vi "Dashboard Main.vi"() -> ()   [LabVIEW 2014]
uses:
  <vilib>/event_ctls.llb/eventvkey.ctl
  <vilib>/Rock Robotics/WPI/Dashboard/WPI_DashboardLogging Global.vi
  <vilib>/Rock Robotics/Network Tables/SD Read Number.vi
  <vilib>/Rock Robotics/Network Tables/SD Write Boolean.vi
  <vilib>/Rock Robotics/Network Tables/SD Write Number.vi
  <vilib>/Utility/config.llb/Write Key (String).vi
  <vilib>/Utility/config.llb/Write Key (I32).vi
  <vilib>/Utility/config.llb/NI_LVConfig.lvlib
panel:
  out "Controls Open 2":bool
  in  "TCP":refnum<k5>
  in  "Rec Mode":enum32{"Stop", "Record", "Playback"}(radio)
  in  "Vision":u16(ring) items=["Camera Off", "USB Camera SW", "USB Camera HW", "IP Camera"]
  out "Camera IP":string
  out "Image Message":string="Timeout in Camera Communications"
  in  "Dashboard Tab":T1(tab)
  in  "?":bool
  in  "?":bool
  in  "Camera Settings":T2={"Frame Rate"=30, "Compression"=30, "Size"=1} {"Frame Rate" scale=1.0..30.0; "Size" items=["640x480", "320x240", "160x120"]}
  out "MotorChart R":cluster{"Numeric":dbl, "Numeric":dbl}(graph)
  out "MotorChart L":T3(graph)
  out "MotorSliders R":cluster{"MotorSlide1":dbl, "MotorSlide2":dbl} {"MotorSlide2" scale=-1.0..1.0 scale format="%#_2e"; "MotorSlide1" scale=-1.0..1.0 scale format="%#_2e"}
  out "MotorSliders L":T4 {"MotorSlide4 2" scale=0.0..14.0 scale format="%#_2e"; "MotorSlide2" scale=-1.0..1.0 scale format="%#_2e"; "MotorSlide1" scale=-1.0..1.0 scale format="%#_2e"}
  out "Gyro":dbl(knob) scale=0.0..360.0
  out "JS1 Z":dbl(slide) scale=-1.0..1.0 scale format="%#_2e"
  out "JS1 Graph":cluster{"X":dbl, "Y":dbl}[](graph)
  out "JS1 Buttons":T5
  out "JS2 Z":dbl(slide) scale=-1.0..1.0 scale format="%#_2e"
  out "JS2 Graph":cluster{"X":dbl, "Y":dbl}[](graph)
  out "JS2 Buttons":T5
  out "Mode":T6(ring)=enum."Auto Disabled"
  in  "DB Camera Config":bool
  out "fps":dbl format="%#.1g"
  out "Mbps":dbl format="%#.1g"
  out "Mbps 2":bool
  in  "DB/String 9":string
  in  "DB/String 8":string
  in  "DB/String 7":string
  in  "DB/String 6":string
  in  "DB/String 5":string
  in  "DB/String 4":string
  in  "DB/String 3":string
  in  "DB/String 2":string
  in  "DB/String 1":string
  in  "DB/String 0":string
  in  "DB/Slider 0":dbl(slide) scale=0.0..5.0
  in  "DB/Slider 1":dbl(slide) scale=0.0..5.0
  in  "DB/Slider 2":dbl(slide) scale=0.0..5.0
  in  "DB/Slider 3":dbl(slide) scale=0.0..5.0
  out "DB/LED 3":bool
  out "DB/LED 2":bool
  out "DB/LED 1":bool
  out "DB/LED 0":bool
  in  "DB/Button 3":bool
  in  "DB/Button 2":bool
  in  "DB/Button 1":bool
  in  "DB/Button 0":bool caption="New Name"
  in  "Auto Encoder Set Point":dbl=10.0
  out "Right Potentiometer":dbl
  out "Left Potentiometer":dbl
  in  "Test Slider":dbl(slide) scale=0.0..100.0 scale format="%#_3g"
  in  "On/Off":bool caption="Solenoid"
  in  "Test Name":u16(ring) items=["Select the test to run...", "Example Test", "-------------------------------", "List of tests is built in robot code.", "Replace with your own automated tests."]
  in  "Test Tree":string(tree)
  in  "Motor":cluster{"Value":dbl, "Enable":bool} {"Value" scale=-1.0..1.0 scale format="%#_3g"}
  out "Progress":T7 {"Test Progress" scale=0.0..100.0}
  in  "Rev/Fwd":cluster{"Forward":bool, "Reverse":bool}
  in  "Test Ring":u16(ring) items=["Monochrome", "Color"]
  in  "Listbox":i32(listbox)
  out "Tree":string(tree)
  out "Camera Image":T8(plugin-control)
  out "Boolean":bool
  out "Controls Open":bool
  # "Left"
  # "Front"
  # "Right"
  # "Battery"
  # "This tab is a great place for autonomous settings and robot-specific values.\nPlace controls and indicators inside this tab and match name to\nDashboard Variables on robot. You can also delete this comment."
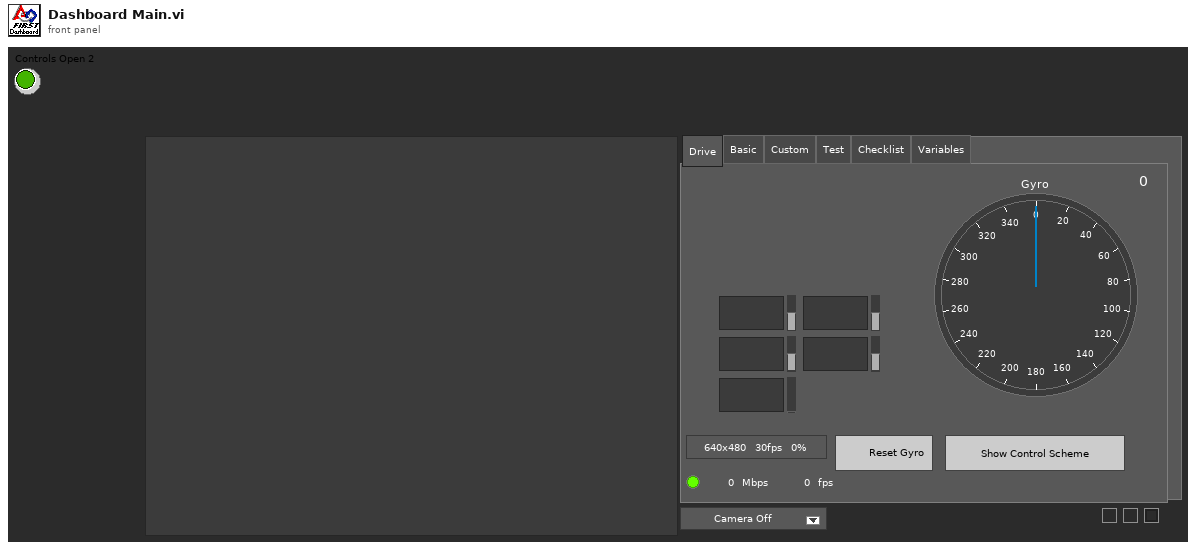
[diagram p1: front panel]
types:
  T1 = enum32{"Drive", "Basic", "Custom", "Test", "Checklist", "Variables"}
  T2 = cluster{"Frame Rate":i32, "Compression":i32, "Size":u16}
  T3 = cluster{"Numeric":dbl, "Numeric":dbl, "Battery V":dbl}
  T4 = cluster{"MotorSlide1":dbl, "MotorSlide2":dbl, "MotorSlide4 2":dbl}
  T5 = cluster{bool, bool, bool, bool, bool, bool, bool, bool, bool, bool, bool, bool}
  T6 = enum8{"Tele-Op Disabled", "Tele-Op Enabled", "Auto Disabled", "Auto Enabled", "Test Disabled", "Test Enabled", "Disconnected", "No Code", "E-Stop"}
  T7 = cluster{"Test Progress":u8, "Test Progress Text":string}
  T8 = typedef "IMAQ Image.ctl" = refnum<image>
  T9 = typedef "Image Type" = u32
  T10 = cluster{"Camera Image":refnum<vi>, "Dashboard Tab":refnum<vi>, "Boolean":refnum<vi>, "Vision":refnum<vi>, "Rec Mode":refnum<vi>, "Test Slider":refnum<vi>, "On/Off ":refnum<vi>, "Test Ring":refnum<vi>, "Rev/Fwd":refnum<vi>, "Test Name":refnum<vi>, "Motor":refnum<vi>, "Progress":refnum<vi>, "CheckList":refnum<vi>, "Tree":refnum<vi>, "Test Tree":refnum<vi>}
  T11 = cluster{"Error Strings":string, "Disable Counts":cluster{u16, u16}, "Rail Faults":cluster{u16, u16, u16}, "Robot IP":string, "DB Mode":u8, "Event Info":cluster{"Name":string, "Type":u8, "Number":u16, "Replay":u8}, "Camera Addr":string}
  T12 = cluster{"Storage":cluster{"Disk Free":u64, "RAM Block":u32, "RAM free":u32}, "CPU Utilization":cluster{"CPU % ISR":sgl, "CPU % Time Crit":sgl, "CPU % Timed Str":sgl, "CPU % High":sgl, "CPU % Above":sgl, "CPU % Normal":sgl, "CPU % Low":sgl}, "CAN":cluster{"% Bus Utilization":sgl, "Bus Off Cnt":u32, "TX_FIFO Full Cnt":u32, "Receive Error Cnt":u8, "Transmit Error Cnt":u8}, "HID":cluster{"HID Outputs":u32, "Rumble Low":u16, "Rumble High":u16}[]}
  T13 = cluster{"Status bits":cluster{"Test Mode":bool, "Autonomous":bool, "Enabled":bool, "Code Start":bool, "Brownout":bool, "Reserved 2":bool, "Reserved 3":bool, "E-Stop":bool}, "Code Trace":cluster{"Disabled":bool, "TeleOp":bool, "Auto":bool, "Test":bool}, "Controller Type":enum16{"unknown", "cRIO", "roboRio"}, "Code?":enum16{"unknown", "noCode", "code"}, "Battery V":dbl}
  T14 = cluster{"Control Bits":cluster{"TestMode":bool, "Autonomous":bool, "Enabled":bool, "FMS Present":bool, bool, bool, bool, "E-Stop":bool}, "Team Station ":u8, "Countdown":sgl, "Joystick Values":cluster{"Axes":dbl[], "Buttons":bool[], "POVs":i16[]}[]}
  T15 = cluster{"Axes":dbl[], "Buttons":bool[], "POVs":i16[]}[]
  T16 = cluster{"Axes":dbl[], "Buttons":bool[], "POVs":i16[]}
  T17 = cluster{"Buttons[0]":bool, "Buttons[1]":bool, "Buttons[2]":bool, "Buttons[3]":bool, "Buttons[4]":bool, "Buttons[5]":bool, "Buttons[6]":bool, "Buttons[7]":bool, "Buttons[8]":bool, "Buttons[9]":bool, "Buttons[10]":bool, "Buttons[11]":bool}
  T18 = typedef "NI_LVConfig.lvlib/Config Data RefNum.ctl" = refnum<k1>
  T19 = cluster{"Operation":enum16{"Update", "Clear"}, "Color Box":u32}[]
  T20 = typedef "eventvkey.ctl" = enum16{"ASCII", "Enter", "Return", "Shift", "Ctrl", "Alt", "Cmd", "Opt", "Caps", "NumLock", "Clear", "Break", "Up", "Down", "Left", "Right", "Insert", "Delete", "Home", "End", "PageUp", "PageDown", "Escape", "Help", "Pause", "ScrollLock", "F1", "F2", "F3", "F4", "F5", "F6", "F7", "F8", "F9", "F10", "F11", "F12", "F13", "F14", "F15", "F16", "F17", "F18", "F19", "F20", "F21", "F22", "F23", "F24", "Play", "VolumeUp", "VolumeDown", "Mute", "Two Byte Char"}
  T21 = cluster{"Image Size":bool, "Image Type":bool, "Pixel Value":bool, "ROI Information":bool, "Zoom Factor":bool}
  T22 = enum8{"Enabled", "Disabled", "Disabled and Grayed Out"}
  T23 = cluster{"Operation":enum16{"Update", "Clear"}, "Color Box":u32}
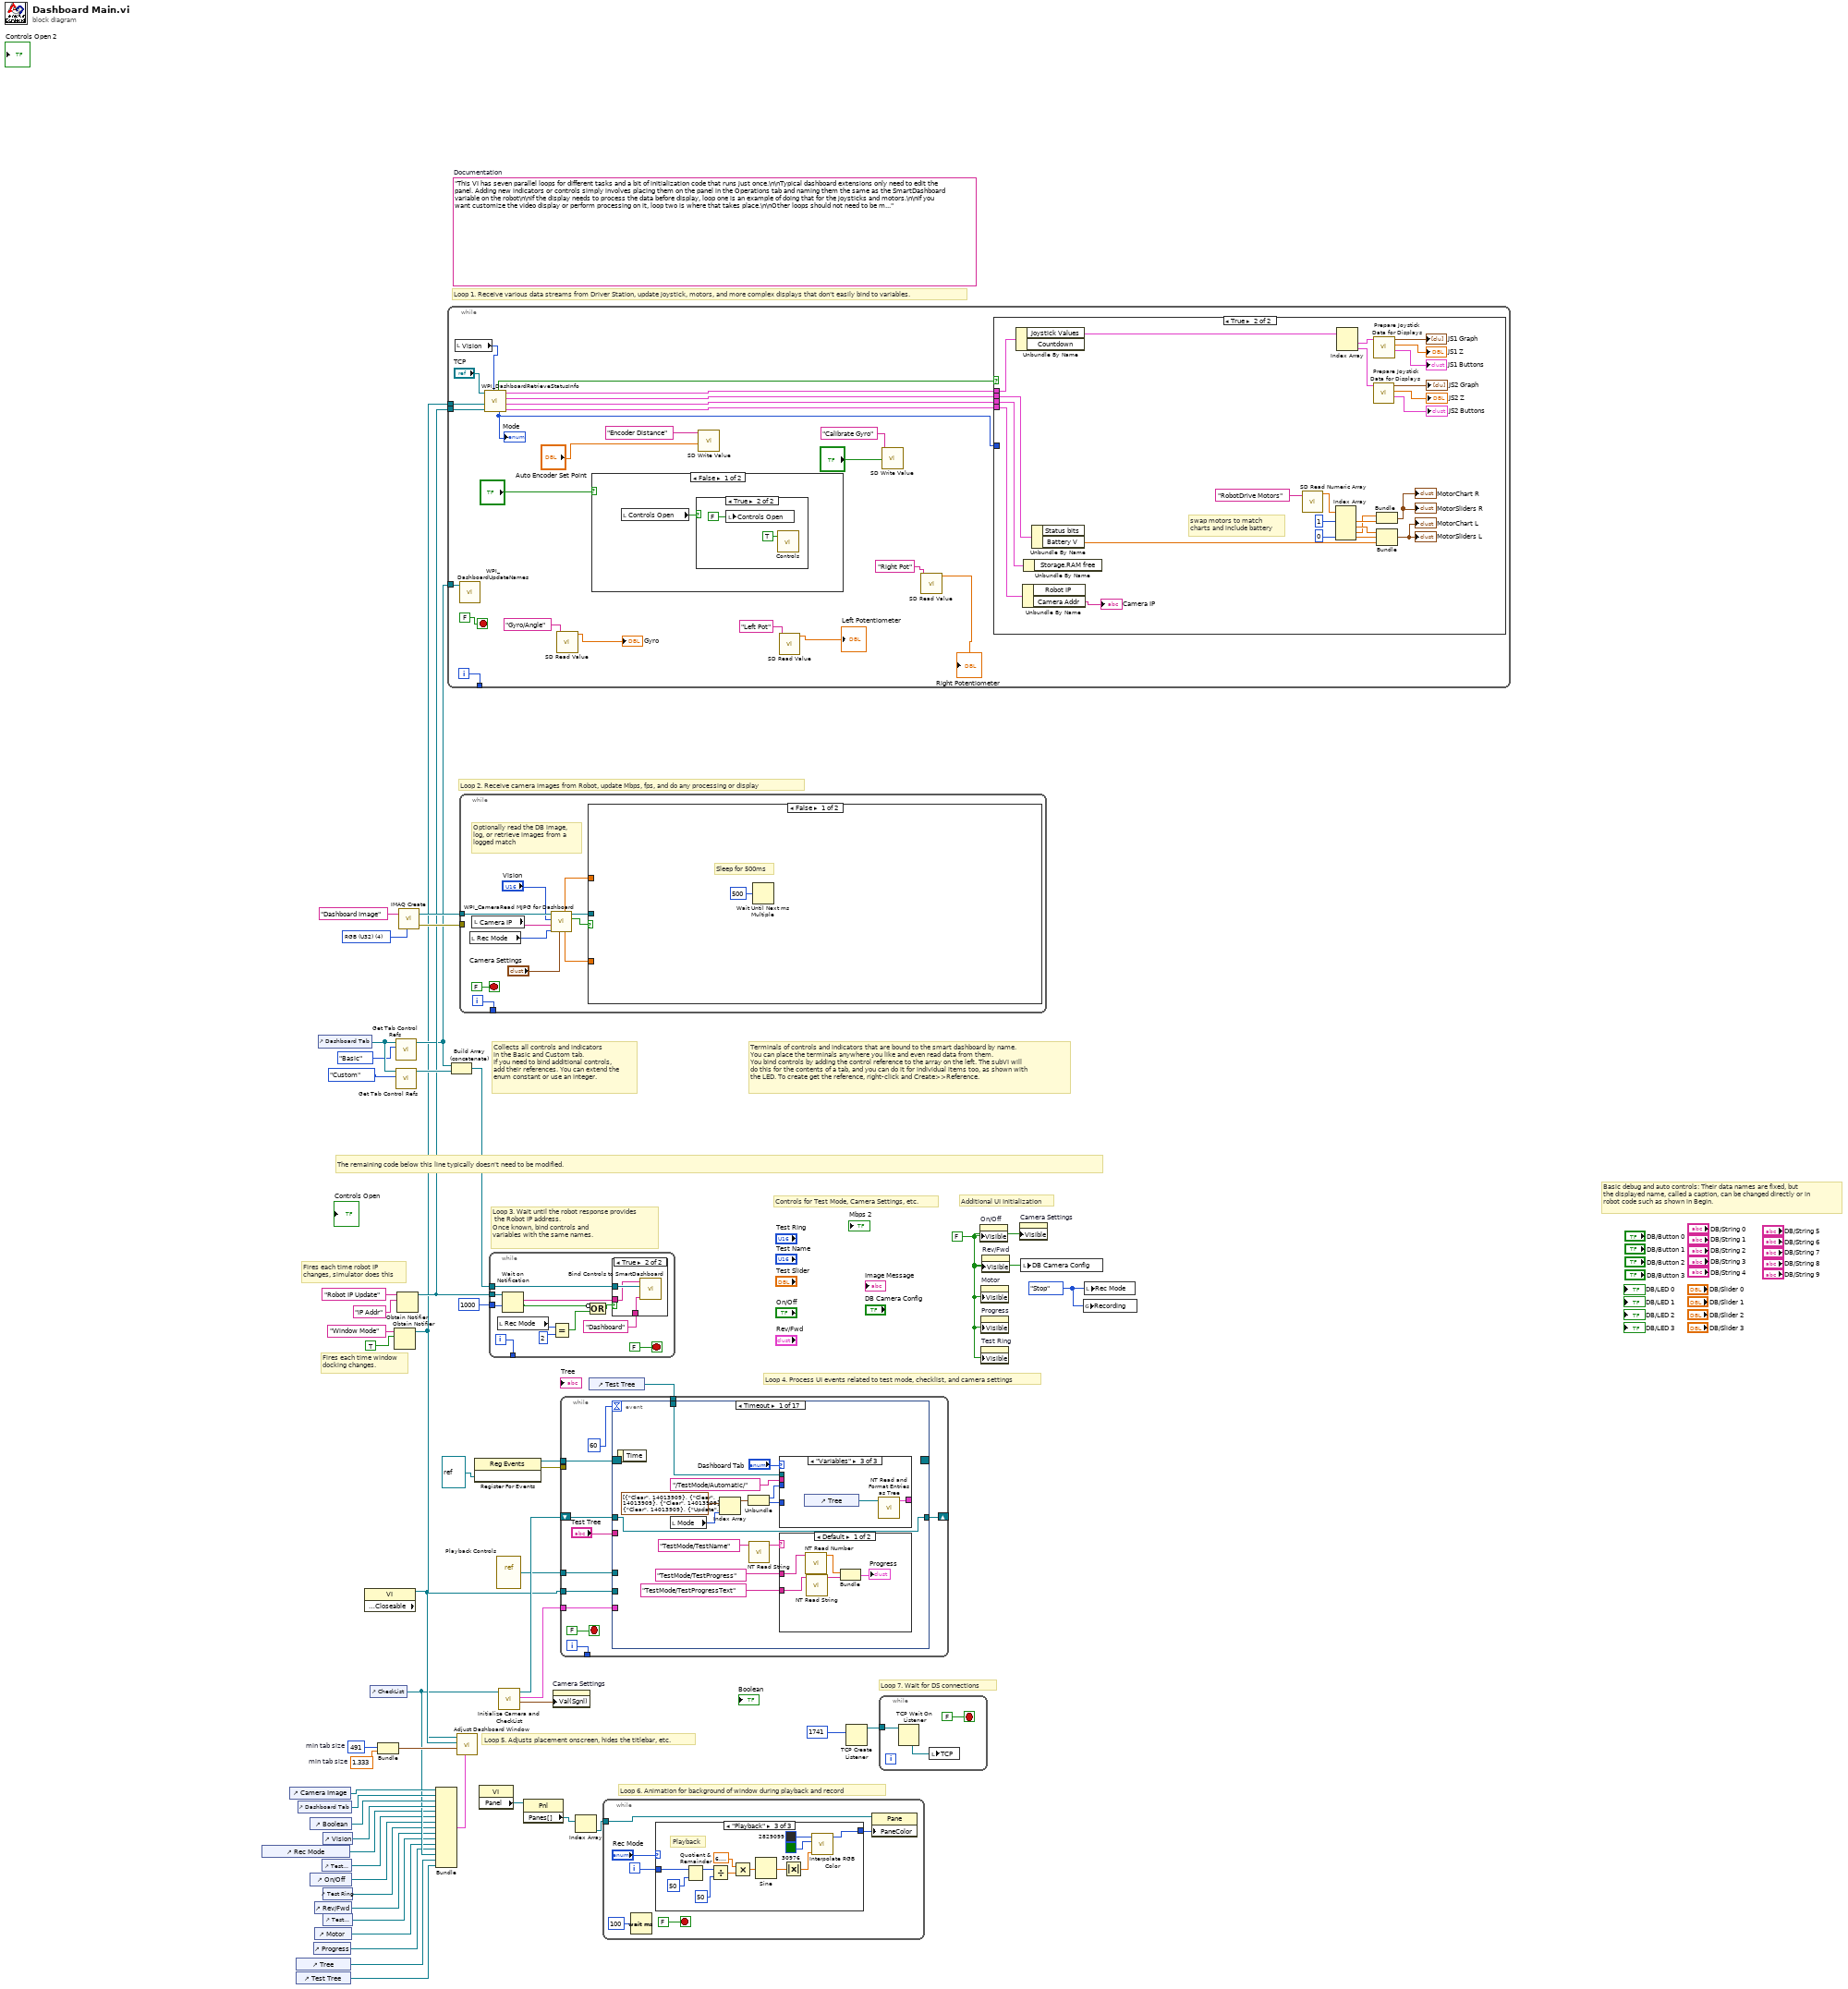
[diagram p0: block diagram]
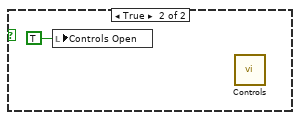
[diagram p3: hidden frame]
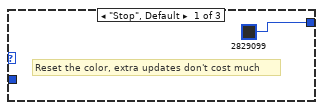
[diagram p5: hidden frame]
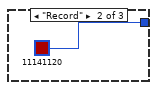
[diagram p6: hidden frame]
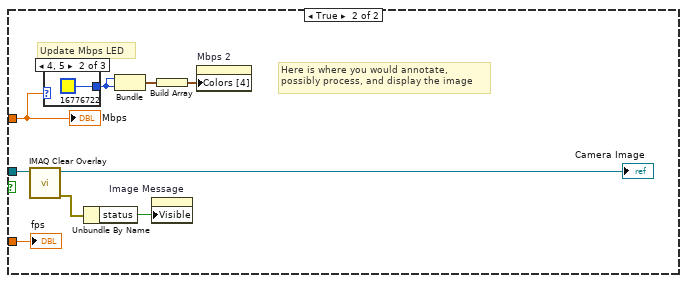
[diagram p8: hidden frame]
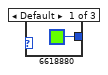
[diagram p9: hidden frame]
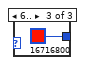
[diagram p10: hidden frame]
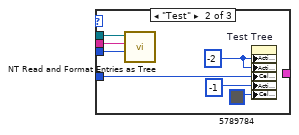
[diagram p12: hidden frame]
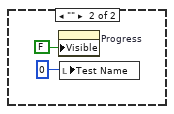
[diagram p13: hidden frame]
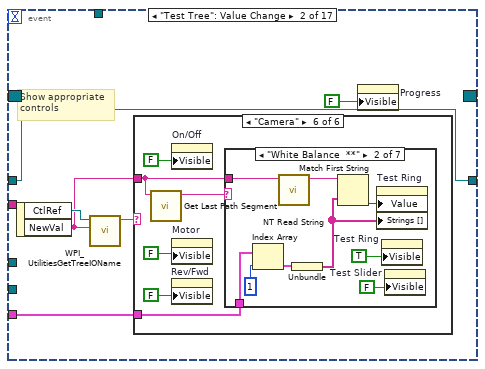
[diagram p14: hidden frame]
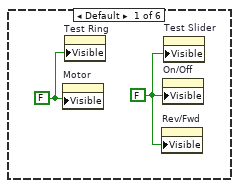
[diagram p15: hidden frame]
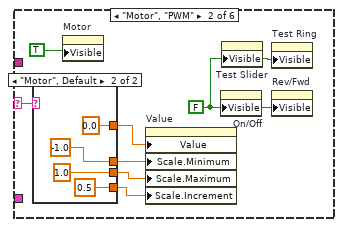
[diagram p16: hidden frame]
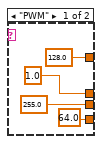
[diagram p17: hidden frame]
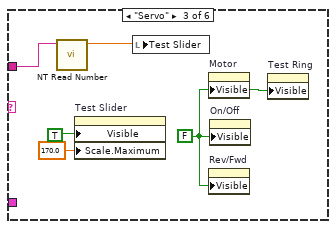
[diagram p18: hidden frame]
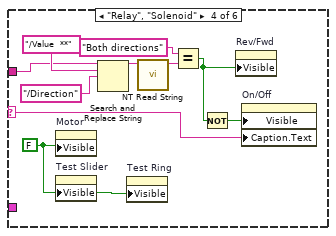
[diagram p19: hidden frame]
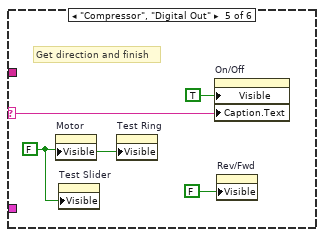
[diagram p20: hidden frame]
diagram:
  w24 = 491  # min tab size
  w23 = 1.333  # min tab size
  w32 = enum32{"Stop", "Record", "Playback"}."Stop" ("Rec Mode")
  w6 = FALSE ("Visible")
  (unwired) "This VI has seven parallel loops for different tasks and a bit of initialization code that runs just once.\n\nTypical dashboard extensions only need to edit the panel. Adding new indicators or controls simply involves placing them on the panel in the Operations tab and naming them the same as the SmartDashboard variable on the robot\n\nIf the display needs to process the data before display, loop one is an example of doing that for the joysticks and motors.\n\nIf you want customize the video display or perform processing on it, loop two is where that takes place.\n\nOther loops should not need to be modified. They are pretty standard, and document the task they perform."  # Documentation
  w52 = T9 4 items=["Grayscale (U8)", "Grayscale (I16)", "Grayscale (SGL)", "Complex (CSG)", "RGB (U32)", "HSL (U32)", "RGB (U64)"] ("Image Type")
  # "Loop 7. Wait for DS connections"
  # "Basic debug and auto controls: Their data names are fixed, but\nthe displayed name, called a caption, can be changed directly or in\nrobot code such as shown in Begin."
  # "Controls for Test Mode, Camera Settings, etc."
  # "Additional UI Initialization"
  # "Loop 6. Animation for background of window during playback and record"
  # "Fires each time robot IP\nchanges, simulator does this"
  # "Fires each time window\ndocking changes."
  # "Collects all controls and indicators\nin the Basic and Custom tab.\nIf you need to bind additional controls,\nadd their references. You can extend the\nenum constant or use an integer."
  # "The remaining code below this line typically doesn't need to be modified."
  # "Loop 4. Process UI events related to test mode, checklist, and camera settings"
  # "Terminals of controls and indicators that are bound to the smart dashboard by name.\nYou can place the terminals anywhere you like and even read data from them.\nYou bind controls by adding the control reference to the array on the left. The subVI will\ndo this for the contents of a tab, and you can do it for individual items too, as shown with\nthe LED. To create get the reference, right-click and Create>>Reference."
  # "Loop 3. Wait until the robot response provides\n the Robot IP address.\nOnce known, bind controls and\nvariables with the same names."
  # "Loop 5. Adjusts placement onscreen, hides the titlebar, etc."
  # "Loop 1. Receive various data streams from Driver Station, update joystick, motors, and more complex displays that don't easily bind to variables."
  # "Loop 2. Receive camera images from Robot, update Mbps, fps, and do any processing or display"
  n1 = control-ref of="Rec Mode"() -> (w12:refnum<vi>)
  n2 = control-ref of="Camera Image"() -> (w27:refnum<vi>)
  n3 = control-ref of="Tree"() -> (w16:refnum<vi>)
  n4 = control-ref of="Test Tree"() -> (w15:refnum<vi>)
  n5 = control-ref of="Dashboard Tab"() -> (w26:refnum<vi>)
  n6 = control-ref of="Boolean"() -> (w21:refnum<vi>)
  n7 = control-ref of="On/Off"() -> (w10:refnum<vi>)
  n8 = control-ref of="Progress"() -> (w7:refnum<vi>)
  n9 = control-ref of="Rev/Fwd"() -> (w8:refnum<vi>)
  n10 = control-ref of="Motor"() -> (w13:refnum<vi>)
  n11 = control-ref of="Dashboard Tab"() -> (w30:refnum<vi>)
  n12 = control-ref of="Test Slider"() -> (w11:refnum<vi>)
  n13 = control-ref of="Vision"() -> (w25:refnum<vi>)
  n14 = control-ref of="Test Ring"() -> (w9:refnum<vi>)
  n15 = control-ref of="Test Name"() -> (w14:refnum<vi>)
  n16 = property class="VI" props=["Front Panel.Closeable"]() -> (reference out=w31:refnum<vi>)  [unwired: 2 in, 2 out]
  n17 = control-ref of="CheckList"() -> (w17:refnum<vi>)
  n18 = Bundle("min tab size"=w24, "min tab size"=w23) -> (w22:cluster{"min tab size":i32, "min tab size":dbl})  [unwired: 1 in]
  n19 = Obtain Notifier(name (unnamed)="Window Mode", notification data type=TRUE) -> (notifier out=w3:refnum<notifier>)  [unwired: 2 in, 2 out]
  n20 = call <vilib>:"Get Tab Control Refs.vi"("Page Index"=T1."Basic" ("Dashboard Tab"), "TabControl in"=w30) -> ("ControlsOnPage"=w4:refnum<vi>[])  [unwired: 9 in]
  n21 = call <vilib>:"Get Tab Control Refs.vi"("Page Index"=T1."Custom" ("Dashboard Tab"), "TabControl in"=w30) -> ("ControlsOnPage"=w29:refnum<vi>[])  [unwired: 9 in]
  n22 = Obtain Notifier(name (unnamed)="Robot IP Update", notification data type="IP Addr" ("name (unnamed)")) -> (notifier out=w5:refnum<notifier>)  [unwired: 2 in, 2 out]
  n23 = call "IMAQ Create"("Image Name"="Dashboard Image", "Image Type"=w52) -> ("New Image"=w50:T8, "error out"=w49:errorcluster)  [unwired: 2 in, 1 out]
  n24 = Bundle("Camera Image"=w27, "Dashboard Tab"=w26, "Boolean"=w21, "Vision"=w25, "Rec Mode"=w12, "Test Slider"=w11, "On/Off"=w10, "Test Ring"=w9, "Rev/Fwd"=w8, "Test Name"=w14, "Motor"=w13, "Progress"=w7, "CheckList"=w17, "Tree"=w16, "Test Tree"=w15) -> (w18:T10)  [unwired: 1 in]
  n25 = while {
    tunnel: [w75] -> _
    tunnel: w5 -> [w69]
    tunnel: w4 -> [w68]
    tunnel: w3 -> [w64]
    i -> [w75]
    stop <- FALSE stop-if-true
    n26 = local read "Vision"() -> (w66:u16)
    n27 = call <vilib>:"WPI_DashboardUpdateNames.vi"("Controls on Tab"=w68) -> ()  [unwired: 11 in]
    n28 = call <vilib>:"WPI_DashboardRetrieveStatusInfo.vi"("Vision"=w66, "Binding Refnum"=w69, "Window Mode Notifier"=w64, "TCP Cnx"="TCP") -> ("Power and Errors"=w70:T11, "Robot Metrics"=w73:T12, "Status Info"=w74:T13, "Control Info"=w71:T14, "Robot Mode"=w67:T6, "Process?"=w72:bool)  [unwired: 2 in]
    "Mode" <- w67
    n29 = call-poly <vilib>:"SD Read Value.vi"("Name"="Gyro/Angle") -> ("Numeric"=→"Gyro":dbl)  [unwired: 8 in, 2 out]
    n30 = case shown="False" "?" {
      frame False {
        n31 = local read "Controls Open"() -> (w77:bool)
        n32 = case shown="True" w77 {
          frame False {
          }
          frame True {
            n33 = local write "Controls Open"(FALSE ("Controls Open")) -> ()
            n34 = call "Controls.vi"("Close"=TRUE) -> ()  [unwired: 11 in]
          }
        }
      }
      frame True {
        n35 = local write "Controls Open"(TRUE) -> ()
        n36 = call "Controls.vi"() -> ()  [unwired: 12 in]
      }
    }
    n37 = call-poly <vilib>:"SD Write Value.vi"("Numeric"="Auto Encoder Set Point", "Name"="Encoder Distance") -> ()  [unwired: 8 in, 2 out]
    n38 = call-poly <vilib>:"SD Read Value.vi"("Name"="Left Pot") -> ("Numeric"=→"Left Potentiometer":dbl)  [unwired: 8 in, 2 out]
    n39 = call-poly <vilib>:"SD Write Value.vi"("Boolean"="?", "Name"="Calibrate Gyro") -> ()  [unwired: 8 in, 2 out]
    n40 = call-poly <vilib>:"SD Read Value.vi"("Name"="Right Pot") -> ("Numeric"=→"Right Potentiometer":dbl)  [unwired: 8 in, 2 out]
    n41 = case shown="True" w72 {
      tunnel: w74 -> [_ w105]
      tunnel: w73 -> [_ w104]
      tunnel: w71 -> [_ w103]
      tunnel: w70 -> [_ w102]
      tunnel: w67 -> [_ _]
      frame False {
      }
      frame True {
        # "swap motors to match\ncharts and include battery"
        n42 = Unbundle By Name(w103) -> ("Joystick Values"=w90:T15)  [unwired: 1 out]
        n43 = Unbundle By Name(w102) -> ("Camera Addr"=→"Camera IP":string)  [unwired: 1 out]
        n44 = Unbundle By Name(w104) -> ()  [unwired: 1 out]
        n45 = Unbundle By Name(w105) -> ("Battery V"=w91:dbl)  [unwired: 1 out]
        n46 = call <vilib>:"SD Read Numeric Array.vi"("Name"="RobotDrive Motors") -> ("Numeric Array"=w93:dbl[])  [unwired: 8 in, 2 out]
        n47 = Index Array(array=w93, index #1=1, index #4=0) -> (element #1=w97:dbl, element #2=w98:dbl, element #3=w96:dbl, element #4=w101:dbl)  [unwired: 2 in]
        n48 = Index Array(array=w90) -> (element #1=w89:T16, element #2=w84:T16)  [unwired: 2 in]
        n49 = call "Prepare Joystick Data for Displays.vi"("Joystick Values"=w84) -> ("Buttons"=→"JS2 Buttons":T17, "Z Axis"=→"JS2 Z":dbl, "Cartesian Data"=→"JS2 Graph":cluster{"X axis":dbl, "X axis":dbl}[])  [unwired: 8 in]
        n50 = call "Prepare Joystick Data for Displays.vi"("Joystick Values"=w89) -> ("Buttons"=→"JS1 Buttons":T17, "Z Axis"=→"JS1 Z":dbl, "Cartesian Data"=→"JS1 Graph":cluster{"X axis":dbl, "X axis":dbl}[])  [unwired: 8 in]
        n51 = Bundle("Numeric"=w96, "Numeric"=w97) -> (→"MotorChart R" →"MotorSliders R":cluster{"Numeric":dbl, "Numeric":dbl})  [unwired: 1 in]
        n52 = Bundle("Numeric"=w98, "Numeric"=w101, "Battery V"=w91) -> (→"MotorChart L" →"MotorSliders L":T3)  [unwired: 1 in]
      }
    }
  }
  n53 = Build Array (concatenate)(w4, w29) -> (w28:refnum<vi>[])
  n54 = call "Adjust Dashboard Window.vi"("Sizing Refnums"=w18, "Size Constraints"=w22, "VI"=w31, "Notifier in"=w3) -> ()  [unwired: 8 in]
  n55 = while {
    tunnel: w50 -> [w114]
    tunnel: w49 -> [_]
    tunnel: [w115] -> _
    i -> [w115]
    stop <- FALSE stop-if-true
    # "Optionally read the DB image,\nlog, or retrieve images from a\nlogged match"
    n56 = local read "Rec Mode"() -> (w108:enum32{"Stop", "Record", "Playback"})
    n57 = local read "Camera IP"() -> (w106:string)
    n58 = call <vilib>:"WPI_CameraRead MJPG for Dashboard.vi"("Camera Settings"="Camera Settings", "Rec Mode"=w108, "Camera IP"=w106, "Camera Mode"="Vision", "Refnum in"=w114) -> ("Active"=w112:bool, "Refnum out"=w113:T8, "FPS"=w111:dbl, "Bandwidth (Mbps)"=w110:dbl)  [unwired: 3 in]
    n59 = case shown="False" w112 {
      tunnel: w113 -> [_ w121]
      tunnel: w110 -> [_ w120]
      tunnel: w111 -> [_ w118]
      frame False {
        # "Sleep for 500ms"
        n60 = Wait Until Next ms Multiple(millisecond multiple=u32 500) -> ()  [unwired: 1 out]
      }
      frame True {
        # "Here is where you would annotate,\npossibly process, and display the image"
        # "Update Mbps LED"
        n61 = call "IMAQ Clear Overlay"("Image"=w121) -> ("error out"=w125:errorcluster, "Image Out"=→"Camera Image":T8)  [unwired: 2 in, 7 out]
        n62 = case shown="4, 5" w120 {
          tunnel: [u32 6618880 ("Color Box") u32 16776722 ("Color Box") u32 16716800 ("Color Box")] -> w122
          frame Default {
          }
          frame 4, 5 {
          }
          frame 6.. {
          }
        }
        n63 = Unbundle By Name(w125) -> ("status"=w126:bool)
        n64 = Bundle("Color Box"=w122, "Color Box"=w122) -> (w124:cluster{"Color Box":u32, "Color Box":u32})  [unwired: 1 out]
        n65 = property on="Image Message" class="Str"("Visible"=w126) -> ()  [unwired: 2 in, 2 out]
        n66 = Build Array(w124) -> (w123:cluster{"Color Box":u32, "Color Box":u32}[])
        n67 = property on="Mbps 2" class="Bool (strict)"("Colors [4]"=w123) -> ()  [unwired: 2 in, 2 out]
        "Mbps" <- w120
        "fps" <- w118
      }
    }
  }
  n68 = register-events(refnum<vi> refnum) -> (reference out=w36:refnum<event-registration>, error out=w35:errorcluster)  [unwired: 2 in]
  n69 = property class="VI"() -> ("Panel"=w39:refnum<vi>)  [unwired: 2 in, 2 out]
  n70 = while {
    tunnel: w28 -> [w141]
    tunnel: w5 -> [w139]
    tunnel: [w137] -> _
    tunnel: u32 1000 ("milliseconds to wait") -> [w136]
    i -> [w137]
    stop <- FALSE stop-if-true
    n71 = local read "Rec Mode"() -> (w132:enum32{"Stop", "Record", "Playback"})
    n72 = Wait on Notification(notifier=w139, timeout in ms (-1)=w136) -> (notification=w138:string, timed out?=w134:bool)  [unwired: 2 in, 2 out]
    n73 = Equal?(x=w132, y=u16 2 ("Rec Mode")) -> (x = y?=w133:bool)
    n74 = Compound Arithmetic op=OR(invert w134, w133) -> (w135:bool)
    n75 = case shown="True" w135 {
      tunnel: w141 -> [_ w144]
      tunnel: w138 -> [_ w143]
      tunnel: "Dashboard" -> [_ w142]
      frame False {
      }
      frame True {
        n76 = call <vilib>:"Bind Controls to SmartDashboard.vi"("Client Name"=w142, "Bound Control Refs"=w144, "Server IP Address"=w143) -> ()  [unwired: 9 in]
      }
    }
  }
  n77 = vi-ref "Playback Controls.vi"() -> (w37:refnum<vi>)
  n78 = call "Initialize Camera and CheckList.vi"("ListBox in"=w17) -> ("Cluster"=w43:cluster{"value":i32, "value":i32, "index":i32}, "Array"=w44:cluster{string[]}[], "File Refnum"=w42:T18)  [unwired: 8 in]
  n79 = property class="Pnl"(reference=w39) -> ("Panes[]"=w40:refnum<vi>[])  [unwired: 1 in, 2 out]
  n80 = property on="Camera Settings" class="Clust (strict)"("Val(Sgnl)"=w43) -> ()  [unwired: 2 in, 2 out]
  n81 = Index Array(array=w40) -> (element=w38:refnum<vi>)  [unwired: 1 in]
  n82 = control-ref of="Test Tree"() -> (w41:refnum<vi>)
  n83 = while {
    tunnel: w44 -> [w152]
    shift-right: [w151] -> _
    shift-left: w42 -> [w150]
    tunnel: [w149] -> _
    tunnel: w41 -> [w148]
    tunnel: w37 -> [w147]
    tunnel: w36 -> [w146]
    tunnel: w35 -> [_]
    tunnel: w31 -> [w145]
    i -> [w149]
    stop <- FALSE stop-if-true
    n84 = event shown="[0] Timeout" {
      selector: w146 -> [_ _ _ _ _ _ _ _ _ _ _ _ _ _ _ _ _]
      dyn-events: [_ _ _ _ _ _ _ _ _ _ _ _ _ w390 _ _ _] -> _
      timeout: u32 60 ("milliseconds to wait") -> [_ _ _ _ _ _ _ _ _ _ _ _ _ _ _ _ _]
      tunnel: w148 -> [w164 _ _ _ _ _ _ _ _ _ _ _ _ _ _ _ _]
      tunnel: "Test Tree" -> [_ _ _ _ _ _ _ _ w359 w367 w369 w373 w381 _ _ _ _]
      tunnel: w152 -> [_ w186 _ _ _ _ w323 w353 _ _ _ _ _ _ _ _ _]
      tunnel: [w160 w185 w284 w289 w297 w309 w322 w346 w358 w365 w368 w372 w380 w392 w406 w407 w417] -> w151
      tunnel: w150 -> [w160 w185 w284 w289 w297 w309 w321 w346 w358 w365 w368 w372 w380 w392 w406 w407 w417]
      tunnel: w147 -> [_ _ _ _ _ _ _ _ _ _ _ _ _ w393 _ w410 _]
      tunnel: w145 -> [_ _ _ _ _ _ _ _ _ _ _ _ _ w388 _ _ _]
      event Timeout {
        n85 = event-data() -> ()  [unwired: 1 in, 1 out]
        n86 = local read "Mode"() -> (w163:T6)
        n87 = Index Array(array=T19 [{"Operation"=enum."Clear", "Color Box"=14013909}, {"Operation"=enum."Clear", "Color Box"=14013909}, {"Operation"=enum."Clear", "Color Box"=14013909}, {"Operation"=enum."Clear", "Color Box"=14013909}, {"Operation"=enum."Update", "Color Box"=14013909}, {"Operation"=enum."Update", "Color Box"=16777215}, {"Operation"=enum."Clear", "Color Box"=14013909}, {"Operation"=enum."Clear", "Color Box"=14013909}, {"Operation"=enum."Clear", "Color Box"=14013909}], index=w163) -> (element=w158:T23)
        n88 = Unbundle(w158) -> ("Operation"=w157:enum16{"Update", "Clear"}, "Color Box"=w156:u32)
        n89 = call <vilib>:"NT Read String.vi"("Name"="TestMode/TestName") -> ("String"=w167:string)  [unwired: 9 in, 1 out]
        n90 = case shown="\"Variables\"" "Dashboard Tab" {
          tunnel: w164 -> [_ w175 _]
          tunnel: "/TestMode/Automatic/" ("Name Pattern") -> [_ w174 _]
          tunnel: w157 -> [_ w173 _]
          tunnel: [_ _ w177] -> _
          tunnel: w156 -> [_ w169 _]
          frame "Custom", Default {
          }
          frame "Test" {
            w172 = -2 ("Active Item:Row Number")
            n91 = call <vilib>:"NT Read and Format Entries as Tree.vi"("Operation"=w173, "Name Pattern"=w174, "Tree Refnum"=w175) -> ()  [unwired: 7 in, 2 out]
            n92 = property on="Test Tree" class="Tree (strict)"("Active Item Row Number"=w172, "ActiveColNum"=w172, "CellBG"=w169, "Active Item Row Number"=-1 ("Active Item:Row Number"), "CellBG"=u32 5789784 ("Color Box")) -> ()  [unwired: 2 in, 2 out]
          }
          frame "Variables" {
            n93 = control-ref of="Tree"() -> (w176:refnum<vi>)
            n94 = call <vilib>:"NT Read and Format Entries as Tree.vi"("Tree Refnum"=w176) -> ("Formatted Strings"=w177:cluster{"Name":string, "Value":string}[])  [unwired: 9 in, 1 out]
          }
        }
        n95 = case shown="Default" w167 {
          tunnel: "TestMode/TestProgress" ("Name") -> [w179 _]
          tunnel: "TestMode/TestProgressText" ("Name") -> [w178 _]
          frame Default {
            n96 = call <vilib>:"NT Read Number.vi"("Name"=w179) -> ("Numeric"=w180:dbl)  [unwired: 9 in, 1 out]
            n97 = call <vilib>:"NT Read String.vi"("Name"=w178) -> ("String"=w181:string)  [unwired: 9 in, 1 out]
            n98 = Bundle("Numeric"=w180, "String"=w181) -> (→"Progress":cluster{"Numeric":dbl, "String":string})  [unwired: 1 in]
          }
          frame "" {
            n99 = property on="Progress" class="Clust (strict)"("Visible"=FALSE) -> ()  [unwired: 2 in, 2 out]
            n100 = local write "Test Name"(u16 0) -> ()
          }
        }
      }
      event "Test Tree": Value Change {
        # "Show appropriate\ncontrols"
        n101 = event-data() -> ("CtlRef"=w189:refnum<vi>, "NewVal"=w187:string)  [unwired: 1 in]
        n102 = call <vilib>:"WPI_UtilitiesGetTreeIOName.vi"("NewVal"=w187, "TreeControl in"=w189) -> ("I/O Name"=w190:string)  [unwired: 9 in]
        n103 = case shown="\"Camera\"" w190 {
          selector: w190 -> [_ w197 _ w215 w224 _]
          tunnel: w187 -> [_ _ w212 w214 _ w231]
          tunnel: w186 -> [_ _ _ _ _ w230]
          frame Default {
            w192 = FALSE ("Visible")
            w191 = FALSE ("Visible")
            n104 = property on="Motor" class="Clust (strict)"("Visible"=w191) -> ()  [unwired: 2 in, 2 out]
            n105 = property on="Test Ring" class="Ring (strict)"("Visible"=w191) -> ()  [unwired: 2 in, 2 out]
            n106 = property on="Rev/Fwd" class="Clust (strict)"("Visible"=w192) -> ()  [unwired: 2 in, 2 out]
            n107 = property on="On/Off" class="Bool (strict)"("Visible"=w192) -> ()  [unwired: 2 in, 2 out]
            n108 = property on="Test Slider" class="Slide (strict)"("Visible"=w192) -> ()  [unwired: 2 in, 2 out]
          }
          frame "Motor", "PWM" {
            w198 = FALSE ("Visible")
            n109 = case shown="\"Motor\", Default" w197 {
              tunnel: [1.0 ("Value") -1.0 ("Value")] -> w196
              tunnel: [255.0 ("Value") 1.0 ("Value")] -> w195
              tunnel: [128.0 ("Value") 0.0 ("Value")] -> w194
              tunnel: [64.0 ("Value") 0.5 ("Value")] -> w193
              frame "PWM" {
              }
              frame "Motor", Default {
              }
            }
            n110 = property on="Motor" class="Clust (strict)"("Visible"=TRUE) -> ()  [unwired: 2 in, 2 out]
            n111 = property on="Value" class="Slide (strict)"("Value"=w194, "Scale.Minimum"=w196, "Scale.Maximum"=w195, "Scale.Increment"=w193) -> ()  [unwired: 2 in, 2 out]
            n112 = property on="On/Off" class="Bool (strict)"("Visible"=w198) -> ()  [unwired: 2 in, 2 out]
            n113 = property on="Test Slider" class="Slide (strict)"("Visible"=w198) -> ()  [unwired: 2 in, 2 out]
            n114 = property on="Test Ring" class="Ring (strict)"("Visible"=w198) -> ()  [unwired: 2 in, 2 out]
            n115 = property on="Rev/Fwd" class="Clust (strict)"("Visible"=w198) -> ()  [unwired: 2 in, 2 out]
          }
          frame "Servo" {
            w210 = FALSE ("Visible")
            n116 = call <vilib>:"NT Read Number.vi"("Name"=w212) -> ("Numeric"=w211:dbl)  [unwired: 9 in, 1 out]
            n117 = property on="Test Slider" class="Slide (strict)"("Visible"=TRUE, "Scale.Maximum"=170.0 ("Scale.Range:Maximum")) -> ()  [unwired: 2 in, 2 out]
            n118 = local write "Test Slider"(w211) -> ()
            n119 = property on="Motor" class="Clust (strict)"("Visible"=w210) -> ()  [unwired: 2 in, 2 out]
            n120 = property on="Rev/Fwd" class="Clust (strict)"("Visible"=w210) -> ()  [unwired: 2 in, 2 out]
            n121 = property on="On/Off" class="Bool (strict)"("Visible"=w210) -> ()  [unwired: 2 in, 2 out]
            n122 = property on="Test Ring" class="Ring (strict)"("Visible"=w210) -> ()  [unwired: 2 in, 2 out]
          }
          frame "Relay", "Solenoid" {
            w213 = FALSE ("Visible")
            n123 = property on="Motor" class="Clust (strict)"("Visible"=w213) -> ()  [unwired: 2 in, 2 out]
            n124 = property on="Test Slider" class="Slide (strict)"("Visible"=w213) -> ()  [unwired: 2 in, 2 out]
            n125 = Search and Replace String(input string=w214, search string="/Value  **", replace string="/Direction") -> (result string=w220:string)  [unwired: 5 in, 3 out]
            n126 = property on="Test Ring" class="Ring (strict)"("Visible"=w213) -> ()  [unwired: 2 in, 2 out]
            n127 = call <vilib>:"NT Read String.vi"("Name"=w220) -> ("String"=w218:string)  [unwired: 9 in, 1 out]
            n128 = Equal?(x="Both directions", y=w218) -> (x = y?=w216:bool)
            n129 = Not(x=w216) -> (.not. x?=w217:bool)
            n130 = property on="Rev/Fwd" class="Clust (strict)"("Visible"=w216) -> ()  [unwired: 2 in, 2 out]
            n131 = property on="On/Off" class="Bool (strict)"("Visible"=w217, "Caption.Text"=w215) -> ()  [unwired: 2 in, 2 out]
          }
          frame "Compressor", "Digital Out" {
            w223 = FALSE ("Visible")
            # "Get direction and finish"
            n132 = property on="Motor" class="Clust (strict)"("Visible"=w223) -> ()  [unwired: 2 in, 2 out]
            n133 = property on="Test Slider" class="Slide (strict)"("Visible"=w223) -> ()  [unwired: 2 in, 2 out]
            n134 = property on="Test Ring" class="Ring (strict)"("Visible"=w223) -> ()  [unwired: 2 in, 2 out]
            n135 = property on="On/Off" class="Bool (strict)"("Visible"=TRUE, "Caption.Text"=w224) -> ()  [unwired: 2 in, 2 out]
            n136 = property on="Rev/Fwd" class="Clust (strict)"("Visible"=FALSE) -> ()  [unwired: 2 in, 2 out]
          }
          frame "Camera" {
            n137 = call <vilib>:"Get Last Path Segment.vi"("String in"=w231) -> ("String out"=w232:string)  [unwired: 10 in]
            n138 = property on="On/Off" class="Bool (strict)"("Visible"=FALSE) -> ()  [unwired: 2 in, 2 out]
            n139 = property on="Motor" class="Clust (strict)"("Visible"=FALSE) -> ()  [unwired: 2 in, 2 out]
            n140 = property on="Rev/Fwd" class="Clust (strict)"("Visible"=FALSE) -> ()  [unwired: 2 in, 2 out]
            n141 = case shown="\"White Balance  **\"" w232 {
              tunnel: w231 -> [w238 w247 w256 w265 w274 _ w280]
              tunnel: w230 -> [w236 w244 w253 w262 w271 _ _]
              frame "Size  **" {
                n142 = Index Array(array=w236) -> (element=w235:cluster{string[]})  [unwired: 1 in]
                n143 = call <vilib>:"NT Read String.vi"("Name"=w238) -> ("String"=w237:string)  [unwired: 9 in, 1 out]
                n144 = Unbundle(w235) -> (w233:string[])
                n145 = Match First String(2:w233, 3:w237) -> (0:w234:i32)  [unwired: 1 out]
                n146 = property on="Test Ring" class="Ring (strict)"("Value"=w234, "Strings []"=w233) -> ()  [unwired: 2 in, 2 out]
                n147 = property on="Test Ring" class="Ring (strict)"("Visible"=TRUE) -> ()  [unwired: 2 in, 2 out]
                n148 = property on="Test Slider" class="Slide (strict)"("Visible"=FALSE) -> ()  [unwired: 2 in, 2 out]
              }
              frame "White Balance  **" {
                n149 = Index Array(array=w244, index=1) -> (element=w245:cluster{string[]})
                n150 = call <vilib>:"NT Read String.vi"("Name"=w247) -> ("String"=w246:string)  [unwired: 9 in, 1 out]
                n151 = Unbundle(w245) -> (w242:string[])
                n152 = Match First String(2:w242, 3:w246) -> (0:w241:i32)  [unwired: 1 out]
                n153 = property on="Test Ring" class="Ring (strict)"("Value"=w241, "Strings []"=w242) -> ()  [unwired: 2 in, 2 out]
                n154 = property on="Test Ring" class="Ring (strict)"("Visible"=TRUE) -> ()  [unwired: 2 in, 2 out]
                n155 = property on="Test Slider" class="Slide (strict)"("Visible"=FALSE) -> ()  [unwired: 2 in, 2 out]
              }
              frame "Exposure  **" {
                n156 = Index Array(array=w253, index=2) -> (element=w254:cluster{string[]})
                n157 = call <vilib>:"NT Read String.vi"("Name"=w256) -> ("String"=w255:string)  [unwired: 9 in, 1 out]
                n158 = Unbundle(w254) -> (w250:string[])
                n159 = Match First String(2:w250, 3:w255) -> (0:w251:i32)  [unwired: 1 out]
                n160 = property on="Test Ring" class="Ring (strict)"("Value"=w251, "Strings []"=w250) -> ()  [unwired: 2 in, 2 out]
                n161 = property on="Test Ring" class="Ring (strict)"("Visible"=TRUE) -> ()  [unwired: 2 in, 2 out]
                n162 = property on="Test Slider" class="Slide (strict)"("Visible"=FALSE) -> ()  [unwired: 2 in, 2 out]
              }
              frame "Exposure Priority  **" {
                n163 = Index Array(array=w262, index=3) -> (element=w263:cluster{string[]})
                n164 = call <vilib>:"NT Read String.vi"("Name"=w265) -> ("String"=w264:string)  [unwired: 9 in, 1 out]
                n165 = Unbundle(w263) -> (w259:string[])
                n166 = Match First String(2:w259, 3:w264) -> (0:w260:i32)  [unwired: 1 out]
                n167 = property on="Test Ring" class="Ring (strict)"("Value"=w260, "Strings []"=w259) -> ()  [unwired: 2 in, 2 out]
                n168 = property on="Test Ring" class="Ring (strict)"("Visible"=TRUE) -> ()  [unwired: 2 in, 2 out]
                n169 = property on="Test Slider" class="Slide (strict)"("Visible"=FALSE) -> ()  [unwired: 2 in, 2 out]
              }
              frame "Color Enable  **" {
                n170 = Index Array(array=w271, index=4) -> (element=w272:cluster{string[]})
                n171 = call <vilib>:"NT Read String.vi"("Name"=w274) -> ("String"=w273:string)  [unwired: 9 in, 1 out]
                n172 = Unbundle(w272) -> (w268:string[])
                n173 = Match First String(2:w268, 3:w273) -> (0:w269:i32)  [unwired: 1 out]
                n174 = property on="Test Ring" class="Ring (strict)"("Value"=w269, "Strings []"=w268) -> ()  [unwired: 2 in, 2 out]
                n175 = property on="Test Ring" class="Ring (strict)"("Visible"=TRUE) -> ()  [unwired: 2 in, 2 out]
                n176 = property on="Test Slider" class="Slide (strict)"("Visible"=FALSE) -> ()  [unwired: 2 in, 2 out]
              }
              frame Default {
                n177 = property on="Test Ring" class="Ring (strict)"("Visible"=FALSE) -> ()  [unwired: 2 in, 2 out]
                n178 = property on="Test Slider" class="Slide (strict)"("Visible"=FALSE) -> ()  [unwired: 2 in, 2 out]
              }
              frame "Brightness  **", "Color Level  **", "Compression  **", "FPS  **", "Sharpness  **" {
                n179 = call <vilib>:"NT Read Number.vi"("Name"=w280) -> ("Numeric"=w279:dbl)  [unwired: 9 in, 1 out]
                n180 = local write "Test Slider"(w279) -> ()
                n181 = property on="Test Slider" class="Slide (strict)"("Visible"=TRUE, "Scale.Maximum"=100.0 ("Scale.Range:Maximum")) -> ()  [unwired: 2 in, 2 out]
                n182 = property on="Test Ring" class="Ring (strict)"("Visible"=FALSE) -> ()  [unwired: 2 in, 2 out]
              }
            }
          }
        }
        n183 = property on="Progress" class="Clust (strict)"("Visible"=FALSE) -> ()  [unwired: 2 in, 2 out]
      }
      event "Test Name": Mouse Enter {
        # "Populate the ring with the list of tests"
        n184 = event-data() -> ()  [unwired: 1 in, 1 out]
        n185 = call <vilib>:"NT Read String Array.vi"("Name"="TestMode/TestList") -> ("String Array"=w288:string[])  [unwired: 9 in, 1 out]
        n186 = Build Array (concatenate)("Select the test to run...", w288) -> (w287:string[])
        n187 = property on="Test Name" class="Ring (strict)"("Strings []"=w287) -> ()  [unwired: 2 in, 2 out]
      }
      event "Test Name": Value Change {
        w290 = FALSE ("Visible")
        # "Tell the robot the test name to run"
        n188 = event-data() -> ("NewVal"=w294:u16)  [unwired: 1 in]
        n189 = property on="Test Name" class="Ring (strict)"() -> ("Strings []"=w295:string[])  [unwired: 2 in, 2 out]
        n190 = local write "Progress"(T7 {"Test Progress"=0, "Test Progress Text"=""} ("Progress")) -> ()
        n191 = Index Array(array=w295, index=w294) -> (element=w293:string)
        n192 = call <vilib>:"NT Write String.vi"("String"=w293, "Name"="TestMode/TestName") -> ()  [unwired: 9 in, 1 out]
        n193 = property on="Progress" class="Clust (strict)"("Visible"=TRUE) -> ()  [unwired: 2 in, 2 out]
        n194 = property on="Motor" class="Clust (strict)"("Visible"=w290) -> ()  [unwired: 2 in, 2 out]
        n195 = property on="Test Slider" class="Slide (strict)"("Visible"=w290) -> ()  [unwired: 2 in, 2 out]
        n196 = property on="On/Off" class="Bool (strict)"("Visible"=w290) -> ()  [unwired: 2 in, 2 out]
        n197 = property on="Rev/Fwd" class="Clust (strict)"("Visible"=w290) -> ()  [unwired: 2 in, 2 out]
        n198 = property on="Test Ring" class="Ring (strict)"("Visible"=w290) -> ()  [unwired: 2 in, 2 out]
      }
      event "Listbox": Double Click {
        # "Shift clears all"
        # "Update symbols on the listbox"
        n199 = event-data() -> ("PlatMods.Shift"=w298:bool, "Row"=w300:i32)  [unwired: 1 in]
        n200 = case shown="True" w298 {
          tunnel: w300 -> [w304 _]
          tunnel: 1 -> [w303 _]
          frame False {
            n201 = property on="Listbox" class="LstBox (strict)"() -> ("Item Symbols"=w302:i32[])  [unwired: 2 in, 2 out]
            n202 = Replace Array Subset(array=w302, new element=w303, index=w304) -> (w301:i32[])
            n203 = property on="Listbox" class="LstBox (strict)"("Item Symbols"=w301) -> ()  [unwired: 2 in, 2 out]
          }
          frame True {
            w305 = 0 ("Top Row")
            n204 = property on="Listbox" class="LstBox (strict)"() -> ("Number of Rows"=w307:u32)  [unwired: 2 in, 2 out]
            n205 = Initialize Array(0, w307) -> (w306:i32[])
            n206 = property on="Listbox" class="LstBox (strict)"("Top Row"=w305, "Value"=w305, "Item Symbols"=w306) -> ()  [unwired: 2 in, 2 out]
          }
        }
      }
      event "Listbox": Key Down {
        # "Update symbols on the listbox\nLeft and right keys check and uncheck"
        n207 = event-data() -> ("VKey"=w311:T20)  [unwired: 1 in]
        n208 = case shown="\"Left\", \"Right\"" w311 {
          selector: w311 -> [w316 _]
          tunnel: eventvkey."Left" ("VKey") -> [w314 _]
          frame "Left", "Right" {
            n209 = Equal?(x=w314, y=w316) -> (x = y?=w315:bool)
            n210 = Select(t=0, s=w315, f=1) -> (s? t:f=w317:i32)
            n211 = property on="Listbox" class="LstBox (strict)"() -> ("Item Symbols"=w320:i32[])  [unwired: 2 in, 2 out]
            n212 = Replace Array Subset(array=w320, new element=w317, index="Listbox") -> (w319:i32[])
            n213 = property on="Listbox" class="LstBox (strict)"("Item Symbols"=w319) -> ()  [unwired: 2 in, 2 out]
          }
          frame Default {
          }
        }
      }
      event "DB Camera Config": Value Change {
        # "Show or hide the cluster of controls, store in ini file"
        n214 = event-data() -> ("NewVal"=w324:bool)  [unwired: 1 in]
        n215 = case shown="False" w324 {
          tunnel: w323 -> [w333 _]
          tunnel: [w326 w344] -> w322
          tunnel: w321 -> [w325 w344]
          frame False {
            w340 = "Camera"
            w343 = FALSE ("Visible")
            n216 = local read "Camera Settings"() -> (w332:T2)
            n217 = Index Array(array=w333) -> (element=w336:cluster{string[]})  [unwired: 1 in]
            n218 = Unbundle(w332) -> ("Frame Rate"=w331:i32, "Compression"=w330:i32, "Size"=w334:u16)
            n219 = Unbundle(w336) -> (w335:string[])
            n220 = Index Array(array=w335, index=w334) -> (element=w329:string)
            n221 = call-poly <vilib>:"Write Key.vi"("section"=w340, "value"=w329, "key"="Size", "refnum"=w325) -> ("refnum out"=w342:T18)  [unwired: 2 in, 5 out]
            n222 = call-poly <vilib>:"Write Key.vi"("section"=w340, "value"=w331, "key"="FrameRate", "refnum"=w342) -> ("refnum out"=w341:T18)  [unwired: 1 in, 6 out]
            n223 = property on="Camera Settings" class="Clust (strict)"("Visible"=w343) -> ()  [unwired: 2 in, 2 out]
            n224 = local write "DB Camera Config"(w343) -> ()
            n225 = call-poly <vilib>:"Write Key.vi"("section"=w340, "value"=w330, "key"="Compression", "refnum"=w341) -> ("refnum out"=w327:T18)  [unwired: 1 in, 6 out]
            n226 = call <vilib>:"Close Config Data.vi"("refnum"=w327) -> ("file path"=w328:path)  [unwired: 2 in, 8 out]
            n227 = call <vilib>:"Open Config Data.vi"("configuration file path"=w328) -> ("refnum"=w326:T18)  [unwired: 8 in, 2 out]
          }
          frame True {
            n228 = property on="Camera Settings" class="Clust (strict)"("Visible"=TRUE) -> ()  [unwired: 2 in, 2 out]
          }
        }
      }
      event "Camera Settings": Value Change {
        # "Update summary string when any elements of DB camera change"
        n229 = event-data() -> ("NewVal"=w357:T2)  [unwired: 1 in]
        n230 = Index Array(array=w353) -> (element=w352:cluster{string[]})  [unwired: 1 in]
        n231 = Unbundle(w357) -> ("Frame Rate"=w348:i32, "Compression"=w347:i32, "Size"=w350:u16)
        n232 = Unbundle(w352) -> (w351:string[])
        n233 = Index Array(array=w351, index=w350) -> (element=w349:string)
        n234 = Format Into String(format string="%s   %dfps   %d%%", w349, w348, w347) -> (resulting string=w354:string)  [unwired: 2 in, 1 out]
        n235 = Build Array(w354) -> (w355:string[])
        n236 = property on="DB Camera Config" class="Bool (strict)"("Strings [4]"=w355) -> ()  [unwired: 2 in, 2 out]
      }
      event "Motor.Enable": Value Change {
        # "When the test mode otor enable helper is set, update that\ntree row item's value"
        n237 = event-data() -> ("NewVal"=w363:bool)  [unwired: 1 in]
        n238 = Unbundle("Motor") -> ("Value"=w362:dbl)  [unwired: 1 out]
        n239 = Select(t=w362, s=w363, f=0.0) -> (s? t:f=w360:dbl)
        n240 = call <vilib>:"NT Write Number.vi"("Numeric"=w360, "Name"=w359) -> ()  [unwired: 9 in, 1 out]
      }
      event "Test Slider": Value Change {
        # "When the test mode slider helper is set, update that\ntree row item's value"
        n241 = event-data() -> ("NewVal"=w366:dbl)  [unwired: 1 in]
        n242 = call <vilib>:"NT Write Number.vi"("Numeric"=w366, "Name"=w367) -> ()  [unwired: 9 in, 1 out]
      }
      event "On/Off": Value Change {
        # "When the test mode on/off helper value is set, update that\ntree row item's value"
        n243 = event-data() -> ("NewVal"=w371:bool)  [unwired: 1 in]
        n244 = Boolean To (0,1)(Boolean=w371) -> (0, 1=w370:i16)
        n245 = call <vilib>:"NT Write Number.vi"("Numeric"=w370, "Name"=w369) -> ()  [unwired: 9 in, 1 out]
      }
      event "Rev/Fwd": Value Change {
        # "When the test mode helper value for relays is set, update that\ntree row item's value"
        n246 = event-data() -> ("NewVal.Forward"=w379:bool, "NewVal.Reverse"=w378:bool)  [unwired: 1 in]
        n247 = Boolean To (0,1)(Boolean=w379) -> (0, 1=w375:i16)
        n248 = Boolean To (0,1)(Boolean=w378) -> (0, 1=w377:i16)
        n249 = Negate(x=w377) -> (-x=w376:i16)
        n250 = Add(x=w375, y=w376) -> (x+y=w374:i16)
        n251 = call <vilib>:"NT Write Number.vi"("Numeric"=w374, "Name"=w373) -> ()  [unwired: 9 in, 1 out]
      }
      event "Test Ring": Value Change {
        # "When a test mode helper value is selected from the ring,\nset the tree item's variable to the string value"
        n252 = event-data() -> ("NewVal"=w383:u16)  [unwired: 1 in]
        n253 = property on="Test Ring" class="Ring (strict)"() -> ("Strings []"=w384:string[])  [unwired: 2 in, 2 out]
        n254 = Index Array(array=w384, index=w383) -> (element=w382:string)
        n255 = call <vilib>:"NT Write String.vi"("String"=w382, "Name"=w381) -> ()  [unwired: 9 in, 1 out]
      }
      event "Rec Mode": Value Change {
        # "Update globals for recording mode and path to read log from.\nClear when logging and let NetworkTables set path for vision to\nuse."
        n256 = event-data() -> ("NewVal"=w394:enum32{"Stop", "Record", "Playback"})  [unwired: 1 in]
        n257 = global write "WPI_DashboardLogging Global.vi" "Logging Filename"(path "") -> ()
        n258 = case shown="\"Playback\"" w394 {
          tunnel: w393 -> [_ w396 w404]
          tunnel: [_ _ w403] -> w390
          tunnel: [_ _ w402] -> _
          tunnel: w388 -> [_ _ w400]
          tunnel: cluster{i32, i32} {-250, 170} -> [_ _ w399]
          tunnel: [_ _ T21 {"Image Size"=TRUE, "Image Type"=TRUE, "Pixel Value"=TRUE, "ROI Information"=TRUE, "Zoom Factor"=FALSE} ("Image Information Shown:All Elements")] -> w386
          tunnel: [_ _ TRUE ("Zoom Factor")] -> w385
          frame Default {
          }
          frame "Stop", "Record" {
            # "Place Window too"
            n259 = invoke class="VI" method="FP.Close"(reference=w396) -> (reference out=w395:refnum<vi>)  [unwired: 2 in, 2 out]
            n260 = invoke class="VI" method="Abort VI"(reference=w395) -> ()  [unwired: 2 in, 3 out]
          }
          frame "Playback" {
            n261 = call "Open Playback Panel.vi"("Offset"=w399, "DB VI Ref"=w400, "Playback in"=w404) -> ("Playback out"=w401:refnum<vi>)  [unwired: 8 in]
            n262 = register-events(w401) -> (reference out=w403:refnum<event-registration>, error out=w402:errorcluster)  [unwired: 2 in]
          }
        }
        n263 = global write "WPI_DashboardLogging Global.vi" "Recording"(w394) -> ()
        n264 = property on="Camera Image" class="ImageControl"("Image Information Shown"=w386, "Image Information Visible"=w385) -> ()  [unwired: 2 in, 2 out]
        n265 = call <vilib>:"WPI_DashboardNT Log FieldName Cache.vi"("Operation"=enum16{"Lookup/Add", "Index", "Clear"}."Clear") -> ()  [unwired: 8 in, 3 out]
      }
      event Panel Close {
        w405 = enum32{"Stop", "Record", "Playback"}."Stop" ("Rec Mode")
        # "Playback window has been closed, abort"
        n266 = event-data() -> ()  [unwired: 1 in, 4 out]
        n267 = local write "Rec Mode"(w405) -> ()
        n268 = global write "WPI_DashboardLogging Global.vi" "Recording"(w405) -> ()
      }
      event Panel Close {
        # "Abort playback window and ourself"
        n269 = event-data() -> ()  [unwired: 1 in, 4 out]
        n270 = invoke class="VI" method="FP.Close"(reference=w410) -> (reference out=w409:refnum<vi>)  [unwired: 2 in, 2 out]
        n271 = invoke class="VI" method="Abort VI"(reference=w409) -> (error out=w408:errorcluster)  [unwired: 2 in, 2 out]
        n272 = invoke class="VI" method="Abort VI"(error in=w408) -> ()  [unwired: 2 in, 3 out]
      }
      event "Vision": Value Change {
        # "Enable/Disable Compression slider.\nHW USB is hard-coded into the camera"
        n273 = event-data() -> ("NewVal"=w416:u16)  [unwired: 1 in]
        n274 = Equal?(x=w416, y=u32 2 ("milliseconds to wait")) -> (x = y?=w414:bool)
        n275 = Select(t=T22."Disabled and Grayed Out" ("Disabled"), s=w414, f=T22."Enabled" ("Disabled")) -> (s? t:f=w411:T22)
        n276 = property on="Compression" class="Slide (strict)"("DisabledEnum"=w411) -> ()  [unwired: 2 in, 2 out]
      }
    }
  }
  n277 = while {
    tunnel: w38 -> [w419]
    i -> [w422]
    stop <- FALSE stop-if-true
    n278 = Wait (ms)(milliseconds to wait=u32 100) -> ()  [unwired: 1 out]
    n279 = case shown="\"Playback\"" "Rec Mode" {
      tunnel: w422 -> [_ _ w437]
      tunnel: [u32 2829099 ("Base Color") u32 11141120 ("Target Color") w426] -> w418
      frame "Stop", Default {
        # "Reset the color, extra updates don't cost much"
      }
      frame "Record" {
      }
      frame "Playback" {
        # "Playback"
        n280 = Quotient & Remainder(x=w437, y=u32 50 ("milliseconds to wait")) -> (x-y*floor(x/y)=w433:u32)  [unwired: 1 out]
        n281 = Divide(x=w433, y=u32 50 ("milliseconds to wait")) -> (x/y=w430:dbl)
        n282 = Multiply(x=6.283185307179586, y=w430) -> (x*y=w435:dbl)
        n283 = Sine(x=w435) -> (sin(x)=w434:dbl)
        n284 = Absolute Value(x=w434) -> (abs(x)=w427:dbl)
        n285 = call "Interpolate RGB Color.vi"("Proportion"=w427, "Target Color"=u32 30976, "Base Color"=u32 2829099) -> ("Result Color"=w426:u32)  [unwired: 8 in]
      }
    }
    n286 = property class="Pane"(reference=w419, "PaneColor"=w418) -> ()  [unwired: 1 in, 2 out]
  }
  n287 = TCP Create Listener(10:u16 1741 ("timeout ms (25000)")) -> (3:w1:refnum<k5>)  [unwired: 4 in, 2 out]
  n288 = while {
    tunnel: w1 -> [w439]
    stop <- FALSE stop-if-true
    n289 = TCP Wait On Listener(11:w439) -> (4:w438:refnum<k5>)  [unwired: 3 in, 4 out]
    n290 = local write "TCP"(w438) -> ()
  }
  n291 = property on="On/Off" class="Bool (strict)"("Visible"=w6) -> ()  [unwired: 2 in, 2 out]
  n292 = property on="Motor" class="Clust (strict)"("Visible"=w6) -> ()  [unwired: 2 in, 2 out]
  n293 = property on="Progress" class="Clust (strict)"("Visible"=w6) -> ()  [unwired: 2 in, 2 out]
  n294 = property on="Test Ring" class="Ring (strict)"("Visible"=w6) -> ()  [unwired: 2 in, 2 out]
  n295 = property on="Rev/Fwd" class="Clust (strict)"("Visible"=w6) -> ()  [unwired: 2 in, 2 out]
  n296 = property on="Camera Settings" class="Clust (strict)"("Visible"=w6) -> ()  [unwired: 2 in, 2 out]
  n297 = local write "DB Camera Config"(w6) -> ()
  n298 = global write "WPI_DashboardLogging Global.vi" "Recording"(w32) -> ()
  n299 = local write "Rec Mode"(w32) -> ()
